vi "SP Scale X Axis.vi"(7 "X-Y Plot":cluster{"X":dbl[], "Y":dbl[]}[](array[cluster]), 8 "error in (no error)":errorcluster, 11 "Plot Reference":refnum<vi>) -> (0 "error out":errorcluster, 3 "Plot Reference":refnum<vi>)   [LabVIEW 2011]
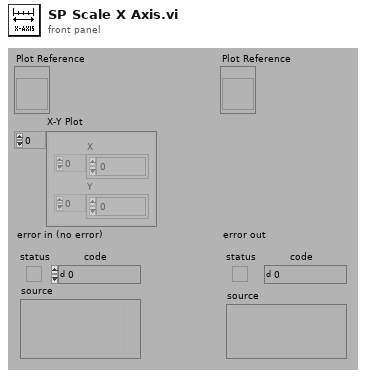
[diagram p1: front panel]
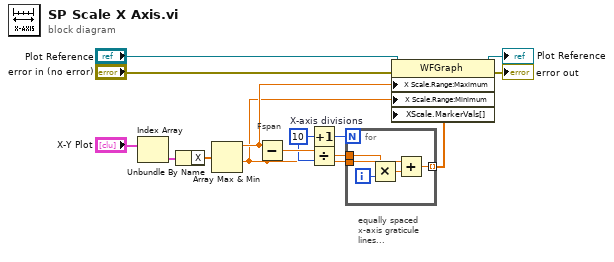
[diagram p0: block diagram]
diagram:
  w6 = 10  # X-axis divisions
  # "equally spaced\nx-axis graticule\nlines..."
  # "Fspan"
  n1 = Index Array(array="X-Y Plot") -> (element=w11:cluster{"X":dbl[], "Y":dbl[]})  [unwired: 1 in]
  n2 = Unbundle By Name(w11) -> ("X"=w8:dbl[])
  n3 = Array Max & Min(array=w8) -> (max value=w5:dbl, min value=w4:dbl)  [unwired: 2 out]
  n4 = Subtract(x=w5, y=w4) -> (x-y=w7:dbl)
  n5 = Increment(x=w6) -> (x+1=w10:i32)
  n6 = Divide(x=w7, y=w6) -> (x/y=w9:dbl)
  n7 = for {
    N: w10 -> [_]
    tunnel: w4 -> [w19]
    tunnel: [w17] -> w3 mode=indexing
    tunnel: w9 -> [w16]
    i -> [w15]
    n8 = Multiply(x=w16, y=w15) -> (x*y=w18:dbl)
    n9 = Add(x=w19, y=w18) -> (x+y=w17:dbl)
  }
  n10 = property on="Property Node" class="WFGraph"(reference="Plot Reference", error in="error in (no error)", "X Scale.Range:Maximum"=w5, "X Scale.Range:Minimum"=w4, "XScale.MarkerVals[]"=w3) -> (reference out=→"Plot Reference":refnum<vi>, error out=→"error out":errorcluster)
